vi "Barcode 1D_Setting_UI.vi"(6 "Analysis_Setting IN":T2={"PreProcess"=enum."*Algorithm*", "Parameter"=""}, 8 "error in (no error)":errorcluster, 9 "ProjectName":string, 10 "ROI List IN":refnum<vi>, 11 "Vision_Image":T9(plugin-control)) -> (0 "error out":errorcluster, 1 "Cancel?":bool, 3 "Analysis_Setting":T2={"PreProcess"=enum."*Algorithm*", "Parameter"=""})   [LabVIEW 2019]
uses:
  <vilib>/userdefined/High Color/IMAQdx.ctl
  <vilib>/vision/NI_Vision_Development_Module.lvlib
  Controls/_UI Command Cluster/Barcode 1D_UI Command Cluster.ctl
  Controls/Analysis_Type.ctl
  Controls/Analysis_Setting.ctl
  Controls/Barcode 1D/Analysis_Barcode 1D_Parameter.ctl
  <vilib>/vision/Instrument.llb/Barcode Search Options.ctl
  Controls/V_Analysis_Type.ctl
  Ctrl/VisionProcessName.ctl
panel:
  in  "Snap?":bool
  in  "Simulaation":bool
  in  "ROI":T1
  out "Numeric":i32
  in  "Done":bool
  in  "Barcode 1D_UI Command":T4(ring)
  in  "Cancel":bool
  in  "Barcode1DTab":T5(tab)
  in  "Barcode Types To Search":u32[](array[ring])=[6, 4, 2] items=["Reserved", "Codabar", "Code 39", "Code 93", "Code 128", "EAN 8", "EAN 13", "Interleaved 2 of 5", "MSI", "UPCA", "Pharmacode", "RSS Limited"]
  in  "Barcode Grading Options":T6={"Calculate Grading Report"=FALSE, "Scan Width "=1}
  in  "Number of Matches Requested":i32=1 min=1 max=9999
  in  "Barcode Search Options":T7={"Min Bar Width"=3, "Min Edge Strength"=75, "Min Bars"=20, "Skip Location Search?"=FALSE}
  out "Barcodes":T8(array[cluster]) {"Confidence Level" format="%.2f"; "Barcode Type" items=["Reserved", "Codabar", "Code 39", "Code 93", "Code 128", "EAN 8", "EAN 13", "Interleaved 2 of 5", "MSI", "UPCA", "Pharmacode", "RSS Limited"]; "Bounding Box"."y" format="%.2f"; "Bounding Box"."x" format="%.2f"}
  # "False"
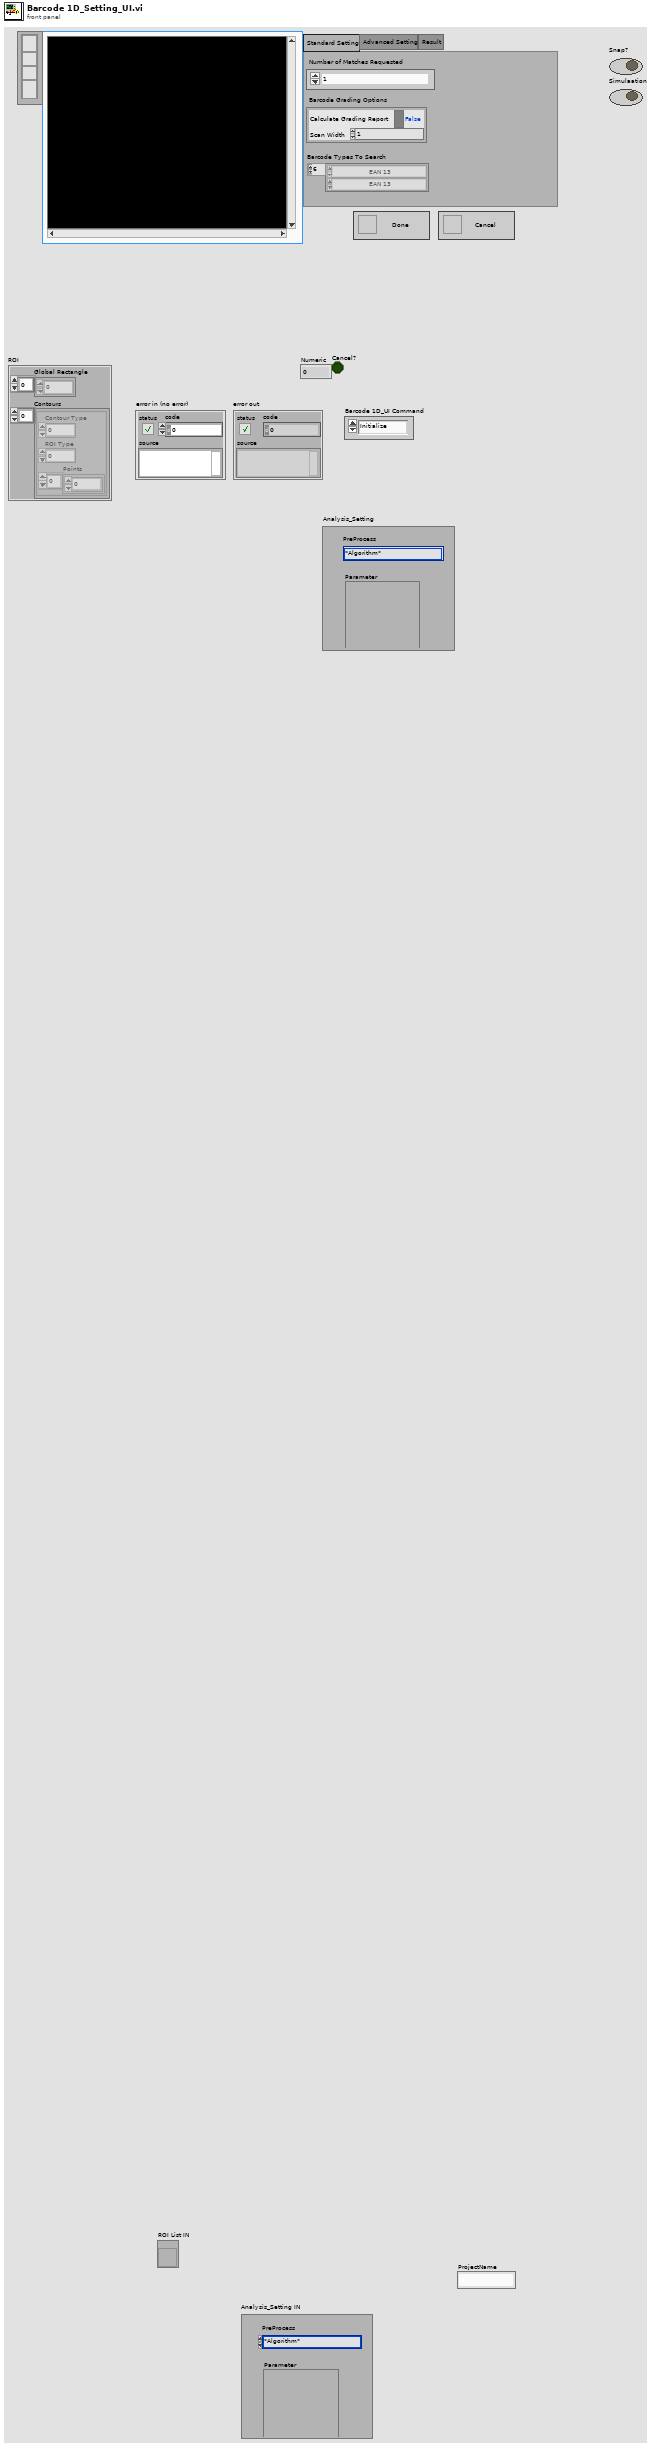
[diagram p1: front panel]
types:
  T1 = cluster{"Global Rectangle":i32[], "Contours":cluster{"Contour Type":u32, "ROI Type":u32, "Points":i32[]}[]}
  T2 = typedef "Analysis_Setting.ctl" = cluster{"PreProcess":T3, "Parameter":string}
  T3 = typedef "VisionProcessName.ctl" = enum16{"*CamParameter*", "CamAttributes", "*Preprocess*", "CG_Brightness", "C_Plane Extraction", "C_Threshold", "G_Lookup Table", "G_Threshold", "B_Image Inversion", "*Algorithm*", "CG_Histogram", "C_Color Matching", "C_Color Pattern Matching", "G_PatternMatch", "CG_Find Straight Edge", "CG_Adv. Find Straight Edge", "CG_Find Circular Edge", "G_Max Clamp", "G_Clamp (Rake)", "G_Pattern Matching"}
  T4 = enum16{"Initialize", "Done", "Run Algorithm", "Cancel"}
  T5 = enum32{"Standard Setting", "Advanced Setting", "Result"}
  T6 = cluster{"Calculate Grading Report":bool, "Scan Width ":i32}
  T7 = typedef "Barcode Search Options.ctl" = cluster{"Min Bar Width":u32, "Min Edge Strength":u32, "Min Bars":u32, "Skip Location Search?":bool}
  T8 = cluster{"Data":string, "Special Char 1":string, "Special Char 2":string, "Checksum(s)":string, "Barcode Type":u32, "Confidence Level":sgl, "Bounding Box":cluster{"x":sgl, "y":sgl}[]}[]
  T9 = typedef "IMAQ Image.ctl" = refnum<image>
  T10 = typedef "Barcode 1D_UI Command Cluster.ctl" = cluster{"Barcode 1D_UI Command":enum16{"Initialize", "Done", "Run Algorithm", "Cancel"}, "Barcode Search Options":T7, "Barcode Types To Search":u32[], "Barcode Grading Options":cluster{"Calculate Grading Report":bool, "Scan Width ":i32}, "Number of Matches Requested":i32, "ROI":cluster{"Global Rectangle":i32[], "Contours":cluster{"Contour Type":u32, "ROI Type":u32, "Points":i32[]}[]}, "Snap Simulation Mouse Down":bool}
  T11 = typedef "IMAQ Line" = cluster{"Start X":i32, "Start Y":i32, "End X":i32, "End Y":i32}
  T12 = typedef "IMAQdx.ctl" = refnum<k21>
  T13 = cluster{"Contour Type":u32, "ROI Type":u32, "Points":i32[]}
  T14 = typedef "Image Type" = u32
  T15 = typedef "Analysis_Barcode 1D_Parameter.ctl" = cluster{"Barcode Search Options":cluster{"Min Bar Width":dbl, "Min Edge Strength":dbl, "Min Bars":dbl, "Skip Location Search?":bool}, "Barcode Types To Search":enum16{"Reserved", "Codabar", "Code 39", "Code 93", "Code 128", "EAN 8", "EAN 13", "Interleaved 2 of 5", "MSI", "UPCA", "Pharmacode", "RSS Limited"}[], "Barcode Grading Options":cluster{"Calculate Grading Report":bool, "Scan Width ":dbl}, "Number of Matches Requested":i32, "ROI":cluster{"Global Rectangle":i32[], "Contours":cluster{"Contour Type":u32, "ROI Type":u32, "Points":i32[]}[]}}
  T16 = typedef "Analysis_Type.ctl" = u16
  T17 = cluster{"Min Bar Width":dbl, "Min Edge Strength":dbl, "Min Bars":dbl, "Skip Location Search?":bool}
  T18 = enum16{"Reserved", "Codabar", "Code 39", "Code 93", "Code 128", "EAN 8", "EAN 13", "Interleaved 2 of 5", "MSI", "UPCA", "Pharmacode", "RSS Limited"}[]
  T19 = cluster{"Calculate Grading Report":bool, "Scan Width ":dbl}
  T20 = typedef "ROI Descriptor" = cluster{"Global Rectangle":i32[], "Contours":cluster{"ID":enum32{"External", "Internal"}, "Type":u32, "Coordinates":i32[]}[]}
  T21 = typedef "Analysis_Setting.ctl" = cluster{"PreProcess":T22, "Parameter":string}
  T22 = typedef "V_Analysis_Type.ctl" = enum16{"None", "C_Color Pattern Matching", "G_PatternMatching", "G_ShapeDectect", "G_GeometricMatch", "B_Area Check"}
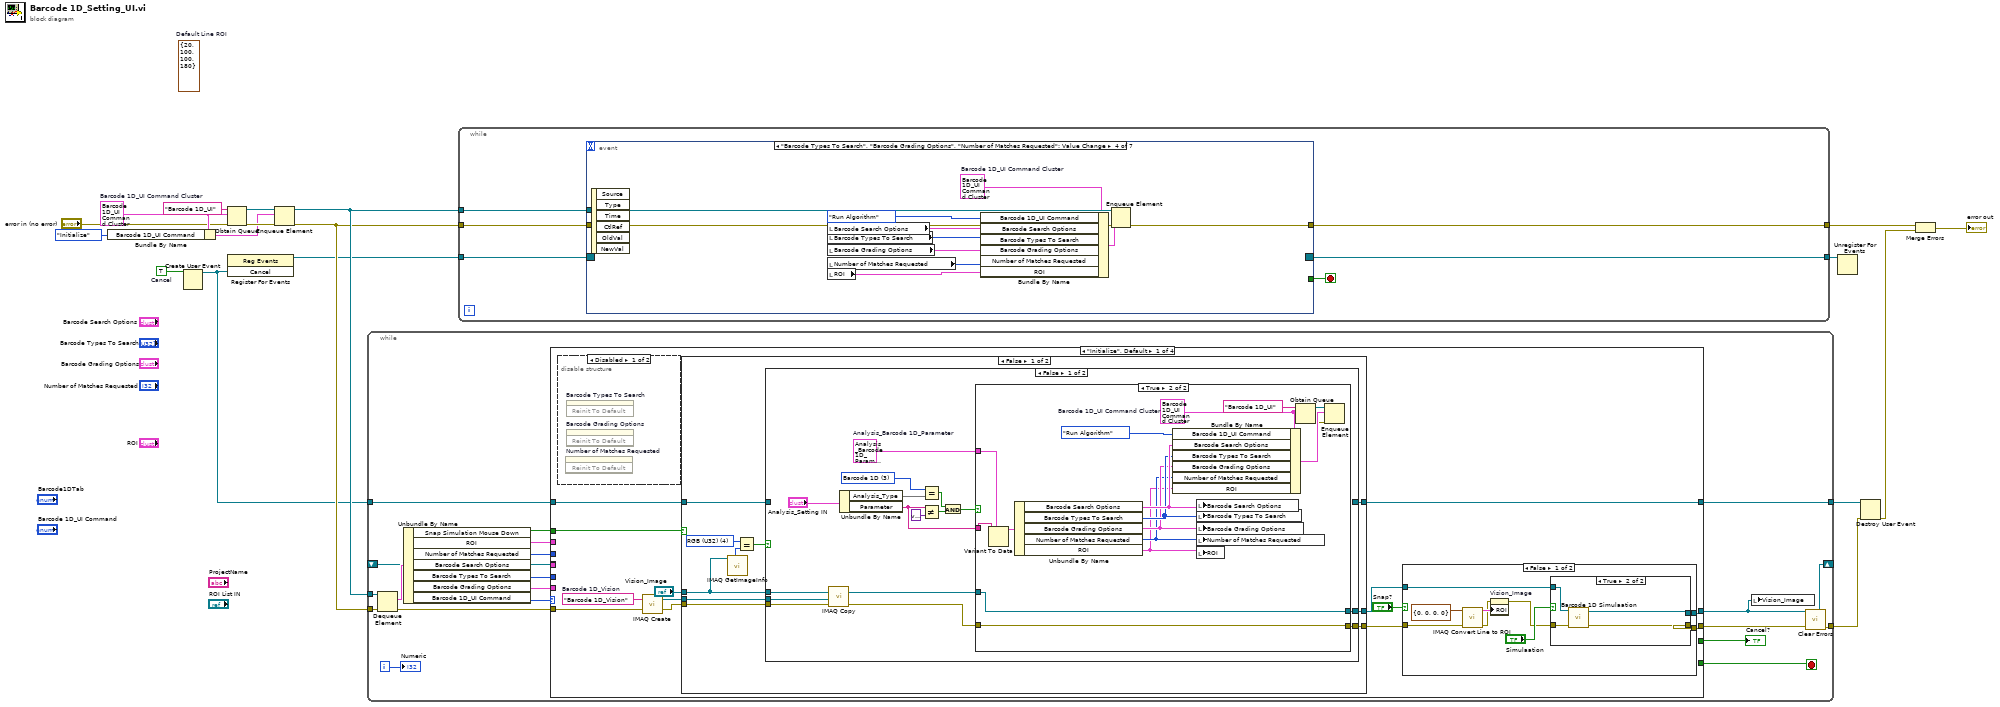
[diagram p0: block diagram]
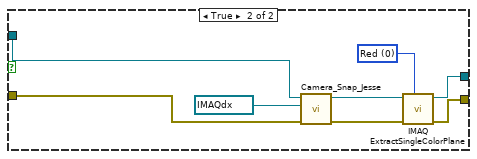
[diagram p4: hidden frame]
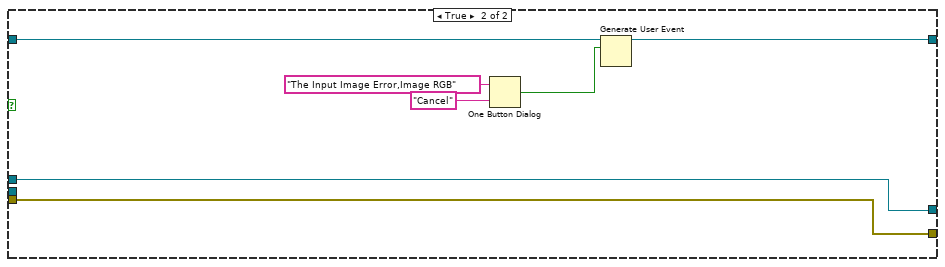
[diagram p6: hidden frame]
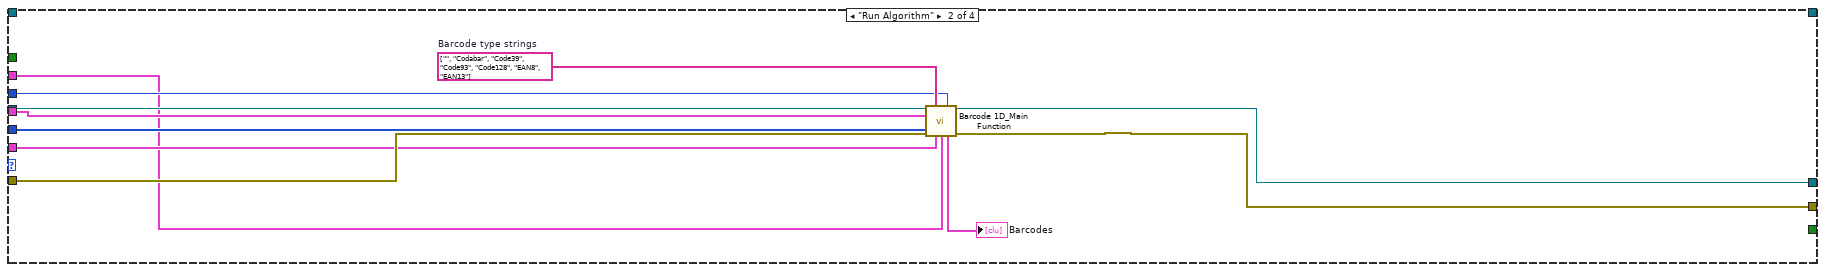
[diagram p8: hidden frame]
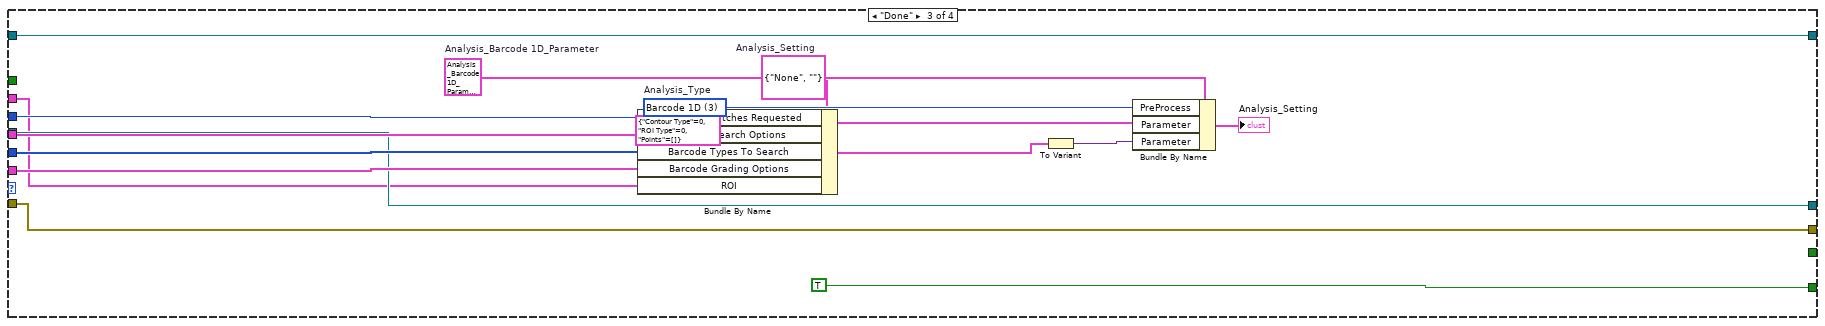
[diagram p9: hidden frame]
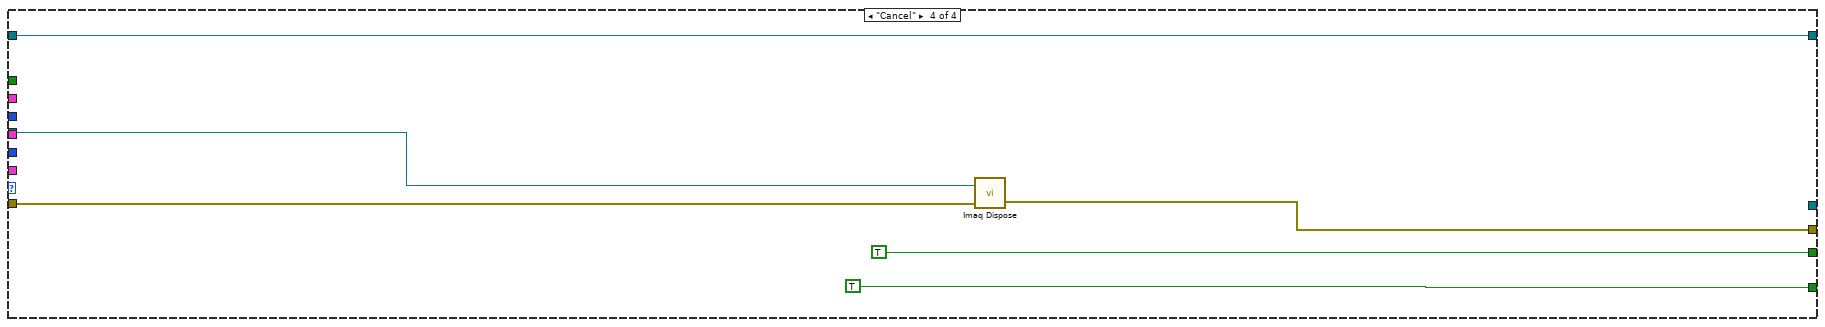
[diagram p10: hidden frame]
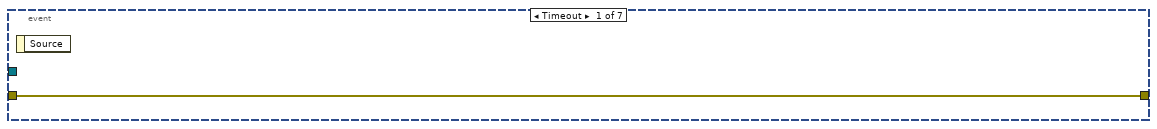
[diagram p11: hidden frame]
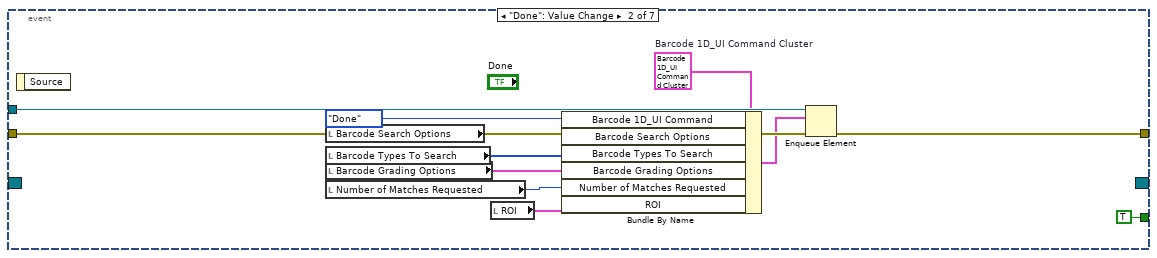
[diagram p12: hidden frame]
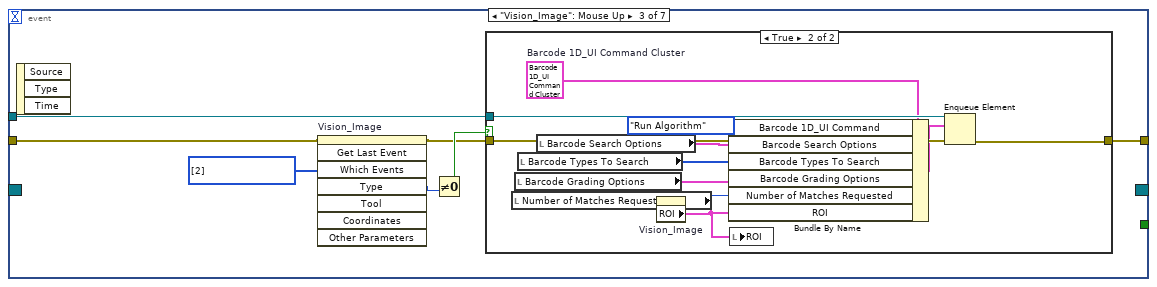
[diagram p13: hidden frame]
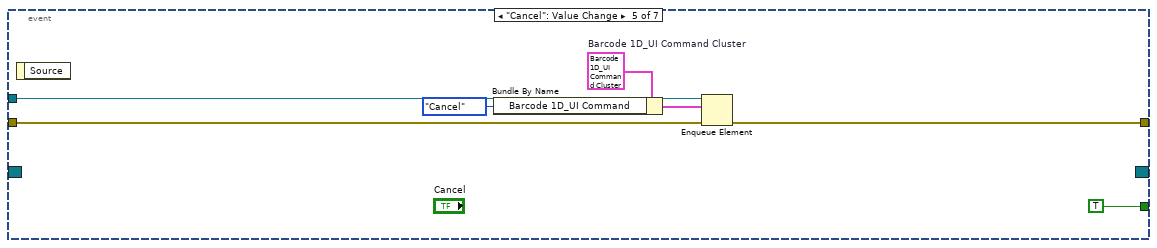
[diagram p15: hidden frame]
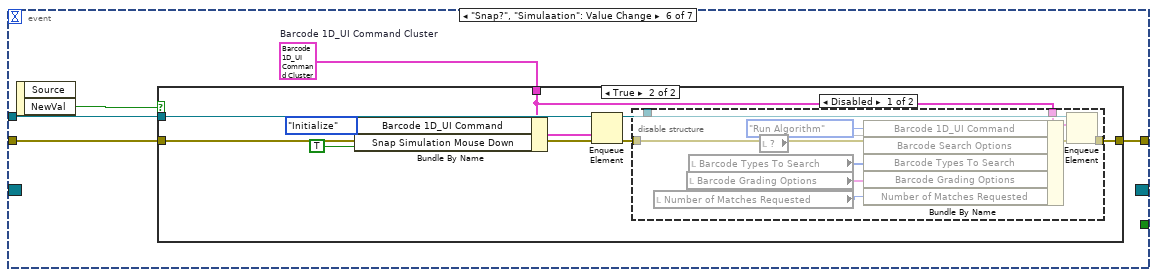
[diagram p16: hidden frame]
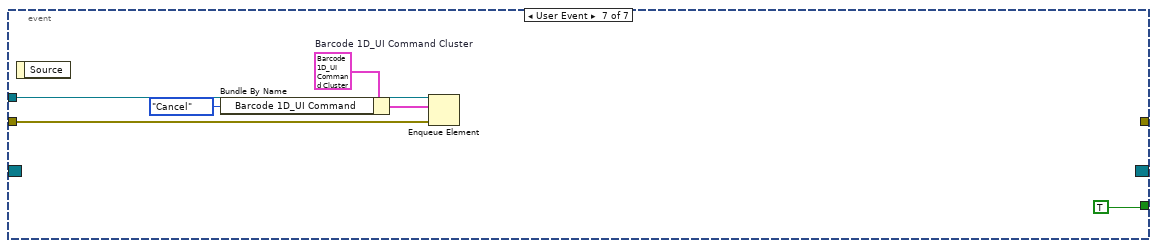
[diagram p19: hidden frame]
diagram:
  w7 = TRUE  # Cancel
  w12 = T10 {"Barcode 1D_UI Command"=enum."Initialize", "Barcode Search Options"={"Min Bar Width"=3, "Min Edge Strength"=75, "Min Bars"=20, "Skip Location Search?"=FALSE}, "Barcode Types To Search"=[6, 4, 2], "Barcode Grading Options"={"Calculate Grading Report"=FALSE, "Scan Width "=1}, "Number of Matches Requested"=1, "ROI"={"Global Rectangle"=[], "Contours"=[]}, "Snap Simulation Mouse Down"=FALSE}  # Barcode 1D_UI Command Cluster
  (unwired) T11 {"Start X"=20, "Start Y"=100, "End X"=100, "End Y"=180}  # Default Line ROI
  n1 = Bundle By Name(cluster=w12, "Barcode 1D_UI Command"=T4."Initialize") -> (w13:T10)
  n2 = Create User Event(user event datatype=w7) -> (user event=w5:refnum<user-event>)  [unwired: 1 in, 1 out]
  n3 = Obtain Queue(name (unnamed)="Barcode 1D_UI", element data type=w12, error in (no error)="error in (no error)") -> (queue out=w18:refnum<queue>, error out=w17:errorcluster)  [unwired: 2 in, 1 out]
  n4 = register-events(w5) -> (reference out=w6:refnum<event-registration>)  [unwired: 2 in, 1 out]
  n5 = Enqueue Element(queue=w18, element=w13, error in (no error)=w17) -> (queue out=w11:refnum<queue>, error out=w10:errorcluster)  [unwired: 1 in, 1 out]
  n6 = while {
    tunnel: w11 -> [w38]
    tunnel: w10 -> [w37]
    shift-right: [w30] -> _
    shift-left: _ -> [w32]
    tunnel: [w20] -> w2
    tunnel: w5 -> [w22]
    tunnel: [w21] -> w4
    i -> [w31]
    stop <- w33 stop-if-true
    n7 = Dequeue Element(queue=w38, error in (no error)=w37) -> (element=w34:T10, error out=w35:errorcluster)  [unwired: 1 in, 2 out]
    n8 = Unbundle By Name(w34) -> ("Snap Simulation Mouse Down"=w23:bool, "ROI"=w24:T1, "Number of Matches Requested"=w25:i32, "Barcode Search Options"=w29:T7, "Barcode Types To Search"=w28:u32[], "Barcode Grading Options"=w27:T6, "Barcode 1D_UI Command"=w36:T4)
    n9 = case shown="\"Initialize\", Default" w36 {
      tunnel: w35 -> [w50 w135 w141 w158]
      tunnel: [w44 w128 w141 w157] -> w19
      tunnel: [_ _ TRUE TRUE] -> w33
      tunnel: [w45 w134 w144 _] -> w30
      tunnel: w32 -> [_ w138 w144 w159]
      tunnel: w29 -> [_ w137 w147 _]
      tunnel: w28 -> [_ w136 w146 _]
      tunnel: w27 -> [_ w133 w145 _]
      tunnel: [_ _ _ TRUE] -> w26
      tunnel: w25 -> [_ w131 w142 _]
      tunnel: w24 -> [_ w129 w140 _]
      tunnel: w23 -> [w49 _ _ _]
      tunnel: w22 -> [w40 _ w139 w155]
      tunnel: [w39 _ w139 w155] -> w21
      frame "Initialize", Default {
        w51 = "Barcode 1D_Vision"  # Barcode 1D_Vision
        n10 = disable-structure shown="Disabled" {
          frame Disabled {
            n11 = invoke on="Number of Matches Requested" class="DigNum (strict)" method="Reinit To Default"() -> ()  [unwired: 3 in, 3 out]
            n12 = invoke on="Barcode Types To Search" class="Arr (strict)" method="Reinit To Default"() -> ()  [unwired: 3 in, 3 out]
            n13 = invoke on="Barcode Grading Options" class="Clust (strict)" method="Reinit To Default"() -> ()  [unwired: 3 in, 3 out]
          }
          frame Enabled {
          }
        }
        n14 = call "IMAQ Create"("Image Name"=w51, "error in (no error)"=w50) -> ("New Image"=w41:T9, "error out"=w42:errorcluster)  [unwired: 3 in]
        n15 = case shown="False" w49 {
          tunnel: [w84 w127] -> w47
          tunnel: [w83 w126] -> w46
          tunnel: w42 -> [w82 w127]
          tunnel: "Vision_Image" -> [w80 _]
          tunnel: w41 -> [w81 w126]
          tunnel: w40 -> [w76 _]
          tunnel: [w75 _] -> w39
          frame False {
            w78 = T14 4 items=["Grayscale (U8)", "Grayscale (I16)", "Grayscale (SGL)", "Complex (CSG)", "RGB (U32)", "HSL (U32)", "RGB (U64)", "Grayscale (U16)"] ("x")
            n16 = call "IMAQ GetImageInfo"("Image"=w80) -> ("Image Type"=w79:T14)  [unwired: 3 in, 7 out]
            n17 = Equal?(x=w78, y=w79) -> (x = y?=w77:bool)
            n18 = case shown="False" w77 {
              tunnel: [w100 w121] -> w84
              tunnel: [w99 w122] -> w83
              tunnel: w82 -> [w89 w121]
              tunnel: w81 -> [w87 _]
              tunnel: w80 -> [w85 w122]
              tunnel: w76 -> [_ w120]
              tunnel: [_ w119] -> w75
              frame False {
                w90 = T15 {"Barcode Search Options"={"Min Bar Width"=0.0, "Min Edge Strength"=0.0, "Min Bars"=0.0, "Skip Location Search?"=FALSE}, "Barcode Types To Search"=[enum."EAN 13", enum."Code 128", enum."Code 39"], "Barcode Grading Options"={"Calculate Grading Report"=FALSE, "Scan Width "=0.0}, "Number of Matches Requested"=1, "ROI"={"Global Rectangle"=[], "Contours"=[]}}  # Analysis_Barcode 1D_Parameter
                w96 = T16 3 items=["None", "PatternMatch", "Edge Detection", "Barcode 1D", "Barcode 2D", "Clamp", "Clamp MAX", "Particle", "Histogram", "Straight Edge", "Circle", "Shape Detect", "OCR", "Contour", "ColorMatch"] ("x")
                n19 = call "IMAQ Copy"("error in (no error)"=w89, "Image Dst"=w87, "Image Src"=w85) -> ("error out"=w86:errorcluster, "Image Dst Out"=w88:T9)  [unwired: 3 in]
                n20 = Unbundle By Name("Analysis_Setting IN") -> ("Analysis_Type"=w95, "Parameter"=w92:string)
                n21 = Not Equal?(x=w92, y=variant) -> (x != y?=w97:bool)
                n22 = Equal?(x=w96, y=w95) -> (x = y?=w98:bool)
                n23 = And(x=w98, y=w97) -> (x .and. y?=w93:bool)
                n24 = case shown="True" w93 {
                  tunnel: w86 -> [w101 w104]
                  tunnel: [w101 w104] -> w100
                  tunnel: [w102 w103] -> w99
                  tunnel: w88 -> [w102 w103]
                  tunnel: w92 -> [_ w118]
                  tunnel: w90 -> [_ w110]
                  frame False {
                  }
                  frame True {
                    w116 = T10 {"Barcode 1D_UI Command"=enum."Initialize", "Barcode Search Options"={"Min Bar Width"=3, "Min Edge Strength"=75, "Min Bars"=20, "Skip Location Search?"=FALSE}, "Barcode Types To Search"=[6, 4, 2], "Barcode Grading Options"={"Calculate Grading Report"=FALSE, "Scan Width "=1}, "Number of Matches Requested"=1, "ROI"={"Global Rectangle"=[], "Contours"=[]}, "Snap Simulation Mouse Down"=FALSE}  # Barcode 1D_UI Command Cluster
                    n25 = Variant To Data(type=w110, Variant=w118) -> (data=w117:T15)  [unwired: 1 in, 1 out]
                    n26 = Unbundle By Name(w117) -> ("Barcode Search Options"=w109:T17, "Barcode Types To Search"=w108:T18, "Barcode Grading Options"=w107:T19, "Number of Matches Requested"=w106:i32, "ROI"=w105:T1)
                    n27 = Bundle By Name(cluster=w116, "Barcode 1D_UI Command"=T4."Run Algorithm", "Barcode Search Options"=w109, "Barcode Types To Search"=w108, "Barcode Grading Options"=w107, "Number of Matches Requested"=w106, "ROI"=w105) -> (w115:T10)
                    n28 = local write "Barcode Search Options"(w109) -> ()
                    n29 = local write "Barcode Types To Search"(w108) -> ()
                    n30 = local write "Barcode Grading Options"(w107) -> ()
                    n31 = local write "Number of Matches Requested"(w106) -> ()
                    n32 = local write "ROI"(w105) -> ()
                    n33 = Obtain Queue(name (unnamed)="Barcode 1D_UI", element data type=w116) -> (queue out=w111:refnum<queue>, error out=w112:errorcluster)  [unwired: 3 in, 1 out]
                    n34 = Enqueue Element(queue=w111, element=w115, error in (no error)=w112) -> ()  [unwired: 1 in, 3 out]
                  }
                }
              }
              frame True {
                n35 = One Button Dialog(message="The Input Image Error,Image RGB", button name ("OK")="Cancel") -> (true=w123:bool)
                n36 = Generate User Event(user event=w120, event data cluster=w123) -> (user event out=w119:refnum<user-event>)  [unwired: 2 in, 1 out]
              }
            }
          }
          frame True {
          }
        }
        n37 = case shown="False" "Snap?" {
          tunnel: [w60 w70] -> w44
          tunnel: [w59 w69] -> w45
          tunnel: w47 -> [w53 w67]
          tunnel: w46 -> [w57 w68]
          frame False {
            n38 = call "IMAQ Convert Line to ROI"("error in (no error)"=w53, "Line"=T11 {"Start X"=0, "Start Y"=0, "End X"=0, "End Y"=0}) -> ("error out"=w54:errorcluster, "ROI Descriptor"=w55:T20)  [unwired: 7 in]
            n39 = property on="Vision_Image" class="ImageControl"(error in=w54, "ROI"=w55) -> (error out=w52:errorcluster)  [unwired: 1 in, 1 out]
            n40 = case shown="True" "Simulaation" {
              tunnel: [w61 w65] -> w60
              tunnel: [w62 w64] -> w59
              tunnel: w52 -> [w61 w66]
              tunnel: w57 -> [w62 w63]
              frame False {
              }
              frame True {
                n41 = call "Barcode 1D Simulaation.vi"("error in (no error)"=w66, "Refnum in"=w63) -> ("error out"=w65:errorcluster, "Refnum out"=w64:T9)  [unwired: 8 in]
              }
            }
          }
          frame True {
            w72 = 0 items=["Red", "Green", "Blue", "Hue", "Saturation", "Luminance", "Value", "Intensity"] ("Color Plane")
            n42 = call "Camera_Snap_Jesse.vi"("error in (no error)"=w67, "Camera Session In"=T12 "cam0", "Image In"=w68) -> ("error out"=w71:errorcluster, "New Image"=w73:T9)  [unwired: 7 in]
            n43 = call "IMAQ ExtractSingleColorPlane"("Color Plane"=w72, "error in (no error)"=w71, "Image Src"=w73) -> ("error out"=w70:errorcluster, "Image Dst Out"=w69:T9)  [unwired: 1 in, 6 out]
          }
        }
      }
      frame "Run Algorithm" {
        w132 = string[] ["", "Codabar", "Code39", "Code93", "Code128", "EAN8", "EAN13"]  # Barcode type strings
        n44 = call "Barcode 1D_Main Function.vi"("Refnum in"=w138, "Barcode type strings IN"=w132, "Number of Matches Requested IN"=w131, "Barcode Search Options IN"=w137, "Barcode Types To Search IN"=w136, "error in (no error)"=w135, "Barcode Grading Options IN"=w133, "ROI Descriptor"=w129) -> ("Refnum out"=w134:T9, "Barcodes"=→"Barcodes":T8, "error out"=w128:errorcluster)  [unwired: 3 in, 2 out]
      }
      frame "Done" {
        w150 = T15 {"Barcode Search Options"={"Min Bar Width"=0.0, "Min Edge Strength"=0.0, "Min Bars"=0.0, "Skip Location Search?"=FALSE}, "Barcode Types To Search"=[enum."EAN 13", enum."Code 128", enum."Code 39"], "Barcode Grading Options"={"Calculate Grading Report"=FALSE, "Scan Width "=0.0}, "Number of Matches Requested"=1, "ROI"={"Global Rectangle"=[], "Contours"=[]}}  # Analysis_Barcode 1D_Parameter
        w152 = T16 3 items=["None", "PatternMatch", "Edge Detection", "Barcode 1D", "Barcode 2D", "Clamp", "Clamp MAX", "Particle", "Histogram", "Straight Edge", "Circle", "Shape Detect", "OCR", "Contour", "ColorMatch"]  # Analysis_Type
        w153 = T21 {"PreProcess"=enum."None", "Parameter"=""}  # Analysis_Setting
        n45 = Bundle By Name(cluster=w150, "Number of Matches Requested"=w142, "Barcode Search Options"=w147, "Barcode Types To Search"=w146, "Barcode Grading Options"=w145, "ROI"=w140) -> (w148:T15)
        n46 = To Variant(anything=w148) -> (Variant=w149:variant)
        n47 = Bundle By Name(cluster=w153, "PreProcess"=w152, "Parameter"=T13 {"Contour Type"=0, "ROI Type"=0, "Points"=[]} ("RegionContour"), "Parameter"=w149) -> (→"Analysis_Setting":T21)
      }
      frame "Cancel" {
        n48 = call "Imaq Dispose"("Image"=w159, "error in (no error)"=w158) -> ("error out"=w157:errorcluster)  [unwired: 4 in]
      }
    }
    "Cancel?" <- w26
    n49 = local write "Vision_Image"(w30) -> ()
    n50 = call <vilib>:"Clear Errors.vi"("error in (no error)"=w19) -> ("error out"=w20:errorcluster)  [unwired: 5 in, 1 out]
    "Numeric" <- w31
  }
  n51 = while {
    tunnel: w11 -> [w166]
    tunnel: w10 -> [w165]
    tunnel: [w163] -> w15
    tunnel: w6 -> [w162]
    tunnel: [w161] -> w3
    stop <- w164 stop-if-true
    n52 = event shown="[3] \"Barcode Types To Search\", \"Barcode Grading Options\", \"Number of Matches Requested\": Value Change" {
      selector: w162 -> [_ _ _ _ _ _ _]
      dyn-events: [_ _ _ _ _ _ _] -> w161
      timeout: _ -> [_ _ _ _ _ _ _]
      tunnel: w166 -> [_ w179 w186 w209 w216 w221 w243]
      tunnel: w165 -> [w167 w178 w183 w208 w215 w220 w242]
      tunnel: [_ TRUE _ _ TRUE _ TRUE] -> w164
      tunnel: [w167 w177 w180 w207 w213 w218 _] -> w163
      event Timeout {
        n53 = event-data() -> ()  [unwired: 1 in, 1 out]
      }
      event "Done": Value Change {
        w176 = T10 {"Barcode 1D_UI Command"=enum."Initialize", "Barcode Search Options"={"Min Bar Width"=3, "Min Edge Strength"=75, "Min Bars"=20, "Skip Location Search?"=FALSE}, "Barcode Types To Search"=[6, 4, 2], "Barcode Grading Options"={"Calculate Grading Report"=FALSE, "Scan Width "=1}, "Number of Matches Requested"=1, "ROI"={"Global Rectangle"=[], "Contours"=[]}, "Snap Simulation Mouse Down"=FALSE}  # Barcode 1D_UI Command Cluster
        n54 = event-data() -> ()  [unwired: 1 in, 1 out]
        n55 = local read "Barcode Search Options"() -> (w170:T7)
        n56 = local read "Barcode Types To Search"() -> (w169:u32[])
        n57 = local read "Barcode Grading Options"() -> (w172:T6)
        n58 = local read "Number of Matches Requested"() -> (w171:i32)
        n59 = local read "ROI"() -> (w168:T1)
        n60 = Bundle By Name(cluster=w176, "Barcode 1D_UI Command"=T4."Done" ("Edge Detection_UI Command"), "Barcode Search Options"=w170, "Barcode Types To Search"=w169, "Barcode Grading Options"=w172, "Number of Matches Requested"=w171, "ROI"=w168) -> (w174:T10)
        n61 = Enqueue Element(queue=w179, element=w174, error in (no error)=w178) -> (error out=w177:errorcluster)  [unwired: 1 in, 2 out]
      }
      event "Vision_Image": Mouse Up {
        w184 = i32[] [2] items=["No Event"=0, "Click Event"=1, "Draw Event"=2, "Size Event"=4, "Scroll Event"=5, "Double Click Event"=8] ("Which Events")
        n62 = event-data() -> ()  [unwired: 1 in, 3 out]
        n63 = invoke on="Vision_Image" class="ImageControl" method="Get Last Event"(error in=w183, "Which Events"=w184) -> (error out=w182:errorcluster, "Type"=w181:i32)  [unwired: 6 in, 6 out]
        n64 = Not Equal To 0?(x=w181) -> (x != 0?=w185:bool)
        n65 = case shown="True" w185 {
          tunnel: w186 -> [_ w197]
          tunnel: w182 -> [w187 w198]
          tunnel: [w187 w196] -> w180
          frame False {
          }
          frame True {
            w195 = T10 {"Barcode 1D_UI Command"=enum."Initialize", "Barcode Search Options"={"Min Bar Width"=3, "Min Edge Strength"=75, "Min Bars"=20, "Skip Location Search?"=FALSE}, "Barcode Types To Search"=[6, 4, 2], "Barcode Grading Options"={"Calculate Grading Report"=FALSE, "Scan Width "=1}, "Number of Matches Requested"=1, "ROI"={"Global Rectangle"=[], "Contours"=[]}, "Snap Simulation Mouse Down"=FALSE}  # Barcode 1D_UI Command Cluster
            n66 = local read "Number of Matches Requested"() -> (w192:i32)
            n67 = local read "Barcode Grading Options"() -> (w191:T6)
            n68 = local read "Barcode Types To Search"() -> (w190:u32[])
            n69 = local read "Barcode Search Options"() -> (w189:T7)
            n70 = property on="Vision_Image" class="ImageControl"() -> ("ROI"=w188:T1)  [unwired: 2 in, 2 out]
            n71 = Bundle By Name(cluster=w195, "Barcode 1D_UI Command"=T4."Run Algorithm", "Barcode Search Options"=w189, "Barcode Types To Search"=w190, "Barcode Grading Options"=w191, "Number of Matches Requested"=w192, "ROI"=w188) -> (w193:T10)
            n72 = local write "ROI"(w188) -> ()
            n73 = Enqueue Element(queue=w197, element=w193, error in (no error)=w198) -> (error out=w196:errorcluster)  [unwired: 1 in, 2 out]
          }
        }
      }
      event "Barcode Types To Search", "Barcode Grading Options", "Number of Matches Requested": Value Change {
        w206 = T10 {"Barcode 1D_UI Command"=enum."Initialize", "Barcode Search Options"={"Min Bar Width"=3, "Min Edge Strength"=75, "Min Bars"=20, "Skip Location Search?"=FALSE}, "Barcode Types To Search"=[6, 4, 2], "Barcode Grading Options"={"Calculate Grading Report"=FALSE, "Scan Width "=1}, "Number of Matches Requested"=1, "ROI"={"Global Rectangle"=[], "Contours"=[]}, "Snap Simulation Mouse Down"=FALSE}  # Barcode 1D_UI Command Cluster
        n74 = event-data() -> ()  [unwired: 1 in, 6 out]
        n75 = local read "Barcode Search Options"() -> (w203:T7)
        n76 = local read "Barcode Types To Search"() -> (w202:u32[])
        n77 = local read "Barcode Grading Options"() -> (w201:T6)
        n78 = local read "Number of Matches Requested"() -> (w200:i32)
        n79 = local read "ROI"() -> (w199:T1)
        n80 = Bundle By Name(cluster=w206, "Barcode 1D_UI Command"=T4."Run Algorithm", "Barcode Search Options"=w203, "Barcode Types To Search"=w202, "Barcode Grading Options"=w201, "Number of Matches Requested"=w200, "ROI"=w199) -> (w205:T10)
        n81 = Enqueue Element(queue=w209, element=w205, error in (no error)=w208) -> (error out=w207:errorcluster)  [unwired: 1 in, 2 out]
      }
      event "Cancel": Value Change {
        w211 = T10 {"Barcode 1D_UI Command"=enum."Initialize", "Barcode Search Options"={"Min Bar Width"=3, "Min Edge Strength"=75, "Min Bars"=20, "Skip Location Search?"=FALSE}, "Barcode Types To Search"=[6, 4, 2], "Barcode Grading Options"={"Calculate Grading Report"=FALSE, "Scan Width "=1}, "Number of Matches Requested"=1, "ROI"={"Global Rectangle"=[], "Contours"=[]}, "Snap Simulation Mouse Down"=FALSE}  # Barcode 1D_UI Command Cluster
        n82 = event-data() -> ()  [unwired: 1 in, 1 out]
        n83 = Bundle By Name(cluster=w211, "Barcode 1D_UI Command"=T4."Cancel") -> (w210:T10)
        n84 = Enqueue Element(queue=w216, element=w210, error in (no error)=w215) -> (error out=w213:errorcluster)  [unwired: 1 in, 2 out]
      }
      event "Snap?", "Simulaation": Value Change {
        w217 = T10 {"Barcode 1D_UI Command"=enum."Initialize", "Barcode Search Options"={"Min Bar Width"=3, "Min Edge Strength"=75, "Min Bars"=20, "Skip Location Search?"=FALSE}, "Barcode Types To Search"=[6, 4, 2], "Barcode Grading Options"={"Calculate Grading Report"=FALSE, "Scan Width "=1}, "Number of Matches Requested"=1, "ROI"={"Global Rectangle"=[], "Contours"=[]}, "Snap Simulation Mouse Down"=FALSE}  # Barcode 1D_UI Command Cluster
        n85 = event-data() -> ("NewVal"=w219:bool)  [unwired: 1 in, 1 out]
        n86 = case shown="True" w219 {
          tunnel: w221 -> [_ w231]
          tunnel: w220 -> [w222 w230]
          tunnel: w217 -> [_ w225]
          tunnel: [w222 w224] -> w218
          frame False {
          }
          frame True {
            n87 = Bundle By Name(cluster=w225, "Barcode 1D_UI Command"=T4."Initialize", "Snap Simulation Mouse Down"=TRUE) -> (w229:T10)
            n88 = Enqueue Element(queue=w231, element=w229, error in (no error)=w230) -> (queue out=w227:refnum<queue>, error out=w226:errorcluster)  [unwired: 1 in, 1 out]
            n89 = disable-structure shown="Disabled" {
              disable-tunnel: w227 -> [w241 _]
              disable-tunnel: w226 -> [w240 _]
              disable-tunnel: w225 -> [w239 _]
              disable-tunnel: [w236 _] -> w224
              frame Disabled {
                n90 = local read "Number of Matches Requested"() -> (w232:i32)
                n91 = local read "Barcode Grading Options"() -> (w233:T6)
                n92 = local read "Barcode Types To Search"() -> (w234:u32[])
                n93 = local read item#-1() -> (w235)
                n94 = Bundle By Name(cluster=w239, "Barcode 1D_UI Command"=T4."Run Algorithm", "Barcode Search Options"=w235, "Barcode Types To Search"=w234, "Barcode Grading Options"=w233, "Number of Matches Requested"=w232) -> (w238:T10)
                n95 = Enqueue Element(queue=w241, element=w238, error in (no error)=w240) -> (error out=w236:errorcluster)  [unwired: 1 in, 2 out]
              }
              frame Enabled {
              }
            }
          }
        }
      }
      event User Event {
        w245 = T10 {"Barcode 1D_UI Command"=enum."Initialize", "Barcode Search Options"={"Min Bar Width"=3, "Min Edge Strength"=75, "Min Bars"=20, "Skip Location Search?"=FALSE}, "Barcode Types To Search"=[6, 4, 2], "Barcode Grading Options"={"Calculate Grading Report"=FALSE, "Scan Width "=1}, "Number of Matches Requested"=1, "ROI"={"Global Rectangle"=[], "Contours"=[]}, "Snap Simulation Mouse Down"=FALSE}  # Barcode 1D_UI Command Cluster
        n96 = event-data() -> ()  [unwired: 1 in, 1 out]
        n97 = Bundle By Name(cluster=w245, "Barcode 1D_UI Command"=T4."Cancel") -> (w244:T10)
        n98 = Enqueue Element(queue=w243, element=w244, error in (no error)=w242) -> ()  [unwired: 1 in, 3 out]
      }
    }
  }
  n99 = Unregister For Events(event registration refnum=w3) -> ()  [unwired: 1 in, 1 out]
  n100 = Destroy User Event(user event=w4, error in=w2) -> (error out=w1:errorcluster)
  n101 = Merge Errors(w15, w1) -> (→"error out":errorcluster)
